vi "TIME_UPLOAD.vi"(8 "error in (no error)":errorcluster, 10 "Cluster":T2={"IP Address"=["", "", "", "", "", "", "", "", "", ""], "Machine name"=["", "", "", "", "", "", "", "", "", ""], "Station number"=["", "", "", "", "", "", "", "", "", ""], "Product List"=[], "Recipe_upload_history path"=path "", "reference"=refnum, "appended array"=[]}, 11 "CtlRef":refnum<vi>) -> (0 "error out":errorcluster, 3 "TIME DATA":i32[](array[numeric]), 5 "Time day":string[](array[string]))   [LabVIEW 2017]
uses:
  Controls/cluster.ctl
  <vilib>/addons/database/Connection.llb/Conn ObjectReference.ctl
  <vilib>/Utility/miscctls.llb/LVDateTimeRec.ctl
  <vilib>/addons/database/NI_Database_API.lvlib
panel:
  out "date time rec":T1
  in  "DAY 1":timestamp format="%<%X\n%x>T"
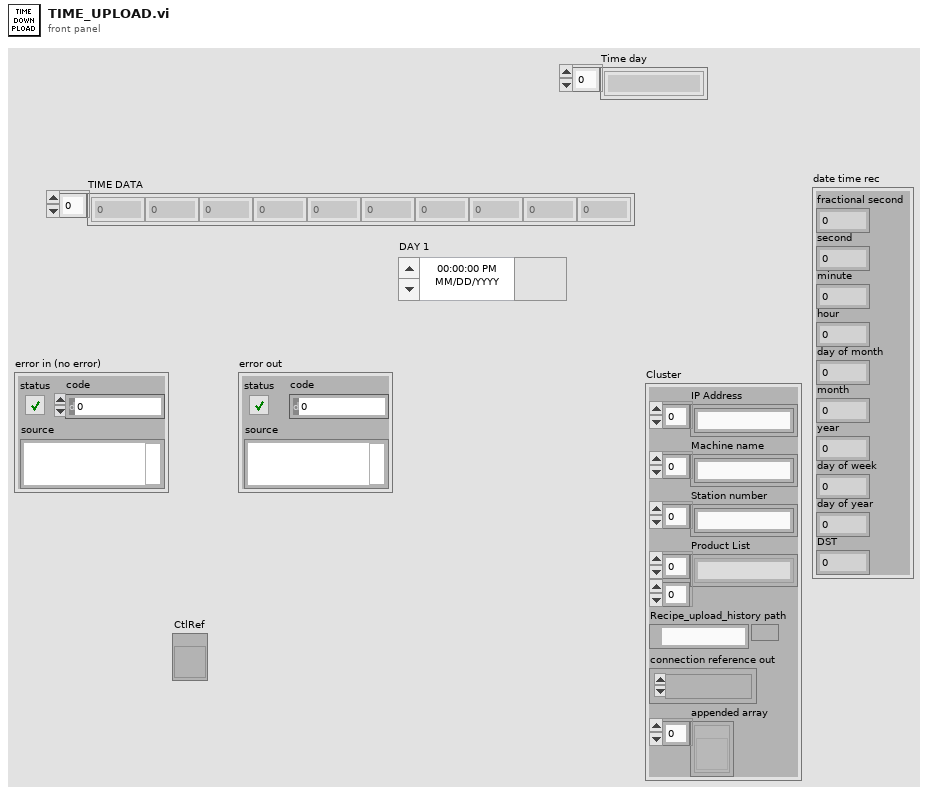
[diagram p1: front panel]
types:
  T1 = typedef "LVDateTimeRec.ctl" = cluster{"fractional second":dbl, "second":i32, "minute":i32, "hour":i32, "day of month":i32, "month":i32, "year":i32, "day of week":i32, "day of year":i32, "DST":i32}
  T2 = typedef "cluster.ctl" = cluster{"IP Address":string[], "Machine name":string[], "Station number":string[], "Product List":string[][], "Recipe_upload_history path":path, "reference":T3, "appended array":refnum<vi>[]}
  T3 = typedef "NI_Database_API.lvlib/Conn ObjectReference.ctl" = refnum<k1>
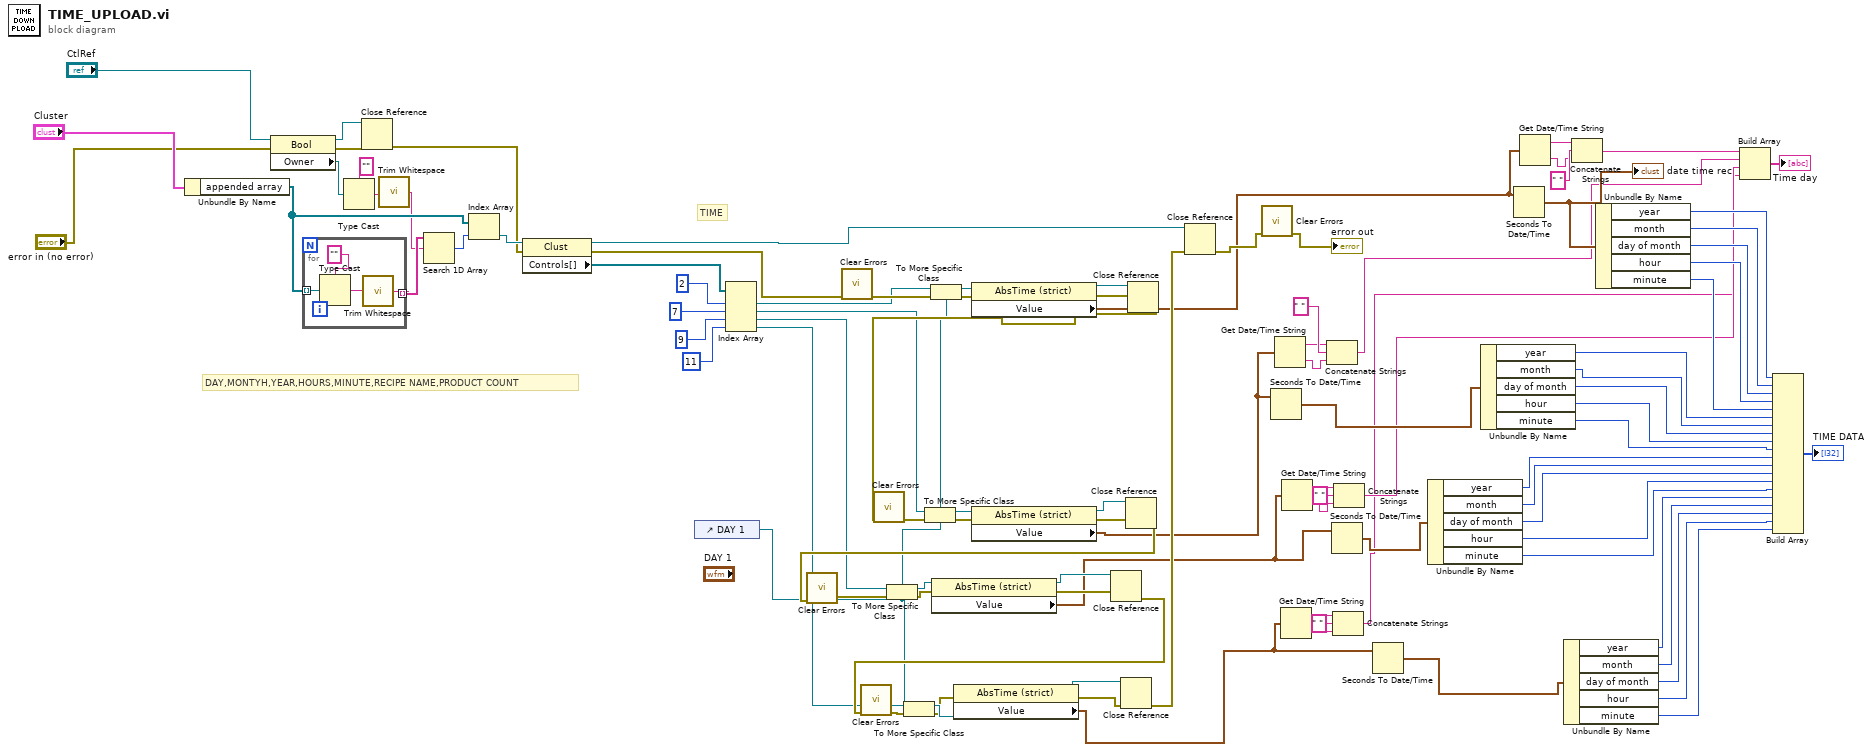
[diagram p0: block diagram]
diagram:
  # "DAY,MONTYH,YEAR,HOURS,MINUTE,RECIPE NAME,PRODUCT COUNT"
  # "TIME"
  n1 = Unbundle By Name("Cluster") -> ("appended array"=w61:refnum<vi>[])
  n2 = property class="Bool"(reference="CtlRef", error in="error in (no error)") -> (reference out=w53:refnum<vi>, error out=w54:errorcluster, "Owner"=w57:refnum<vi>)
  n3 = for {
    tunnel: w61 -> [w102] mode=indexing
    tunnel: [w99] -> w59 mode=indexing
    n4 = Type Cast(type="" ("String"), x=w102) -> (*(type *) &x=w100:string)
    n5 = call <vilib>:"Trim Whitespace.vi"("string"=w100) -> ("trimmed string"=w99:string)  [unwired: 1 in]
  }
  n6 = Type Cast(type="", x=w57) -> (*(type *) &x=w56:string)
  n7 = Close Reference(reference=w53, error in (no error)=w54) -> (error out=w49:errorcluster)
  n8 = call <vilib>:"Trim Whitespace.vi"("string"=w56) -> ("trimmed string"=w58:string)  [unwired: 1 in]
  n9 = Search 1D Array(1D array=w59, element=w58) -> (index of element=w60:i32)  [unwired: 1 in]
  n10 = Index Array(array=w61, index=w60) -> (element=w50:refnum<vi>)
  n11 = property class="Clust"(reference=w50, error in=w49) -> (reference out=w96:refnum<vi>, error out=w97:errorcluster, "Controls[]"=w94:refnum<vi>[])
  n12 = control-ref of="DAY 1"() -> (w63:refnum<vi>)
  n13 = Index Array(array=w94, index #1=2 ("index"), index #2=7 ("index"), index #3=9 ("index"), index #4=11 ("index")) -> (element #1=w67:refnum<vi>, element #2=w71:refnum<vi>, element #3=w76:refnum<vi>, element #4=w83:refnum<vi>)
  n14 = call <vilib>:"Clear Errors.vi"("error in (no error)"=w97) -> ("error out"=w70:errorcluster)  [unwired: 5 in, 1 out]
  n15 = To More Specific Class(target class=w63, reference=w67, error in=w70) -> (specific class reference=w68:refnum<vi>, error out=w69:errorcluster)
  n16 = property class="AbsTime (strict)"(reference=w68, error in=w69) -> (reference out=w86:refnum<vi>, error out=w95:errorcluster, "Value"=w21:timestamp)
  n17 = Close Reference(reference=w86, error in (no error)=w95) -> (error out=w89:errorcluster)
  n18 = call <vilib>:"Clear Errors.vi"("error in (no error)"=w89) -> ("error out"=w74:errorcluster)  [unwired: 5 in, 1 out]
  n19 = To More Specific Class(target class=w63, reference=w71, error in=w74) -> (specific class reference=w72:refnum<vi>, error out=w73:errorcluster)
  n20 = property class="AbsTime (strict)"(reference=w72, error in=w73) -> (reference out=w85:refnum<vi>, error out=w92:errorcluster, "Value"=w15:timestamp)
  n21 = Close Reference(reference=w85, error in (no error)=w92) -> (error out=w88:errorcluster)
  n22 = call <vilib>:"Clear Errors.vi"("error in (no error)"=w88) -> ("error out"=w77:errorcluster)  [unwired: 5 in, 1 out]
  n23 = To More Specific Class(target class=w63, reference=w76, error in=w77) -> (specific class reference=w75:refnum<vi>, error out=w78:errorcluster)
  n24 = property class="AbsTime (strict)"(reference=w75, error in=w78) -> (reference out=w84:refnum<vi>, error out=w91:errorcluster, "Value"=w12:timestamp)
  n25 = Close Reference(reference=w84, error in (no error)=w91) -> (error out=w87:errorcluster)
  n26 = call <vilib>:"Clear Errors.vi"("error in (no error)"=w87) -> ("error out"=w80:errorcluster)  [unwired: 5 in, 1 out]
  n27 = To More Specific Class(target class=w63, reference=w83, error in=w80) -> (specific class reference=w81:refnum<vi>, error out=w79:errorcluster)
  n28 = property on="Property Node" class="AbsTime (strict)"(reference=w81, error in=w79) -> (reference out=w82:refnum<vi>, error out=w62:errorcluster, "Value"=w10:timestamp)
  n29 = Close Reference(reference=w82, error in (no error)=w62) -> (error out=w90:errorcluster)
  n30 = Close Reference(reference=w96, error in (no error)=w90) -> (error out=w47:errorcluster)
  n31 = call <vilib>:"Clear Errors.vi"("error in (no error)"=w47) -> ("error out"=→"error out":errorcluster)  [unwired: 5 in, 1 out]
  n32 = Seconds To Date/Time(time stamp (now)=w15) -> (date time rec=w40:T1)  [unwired: 1 in]
  n33 = Get Date/Time String(seconds (now)=w15) -> (date string=w4:string, time string=w17:string)  [unwired: 2 in]
  n34 = Get Date/Time String(seconds (now)=w10) -> (date string=w2:string, time string=w1:string)  [unwired: 2 in]
  n35 = Get Date/Time String(seconds (now)=w12) -> (date string=w3:string, time string=w13:string)  [unwired: 2 in]
  n36 = Concatenate Strings(w4, " " ("string"), w17) -> (w8:string)
  n37 = Seconds To Date/Time(time stamp (now)=w12) -> (date time rec=w34:T1)  [unwired: 1 in]
  n38 = Concatenate Strings(w2, " " ("string"), w1) -> (w6:string)
  n39 = Concatenate Strings(w3, " " ("string"), w13) -> (w7:string)
  n40 = Seconds To Date/Time(time stamp (now)=w10) -> (date time rec=w28:T1)  [unwired: 1 in]
  n41 = Unbundle By Name(w34) -> ("year"=w33:i32, "month"=w32:i32, "day of month"=w31:i32, "hour"=w30:i32, "minute"=w29:i32)
  n42 = Unbundle By Name(w40) -> ("year"=w39:i32, "month"=w38:i32, "day of month"=w37:i32, "hour"=w36:i32, "minute"=w35:i32)
  n43 = Seconds To Date/Time(time stamp (now)=w21) -> (date time rec=w22:T1)  [unwired: 1 in]
  "date time rec" <- w22
  n44 = Get Date/Time String(seconds (now)=w21) -> (date string=w20:string, time string=w18:string)  [unwired: 2 in]
  n45 = Unbundle By Name(w28) -> ("year"=w27:i32, "month"=w26:i32, "day of month"=w25:i32, "hour"=w24:i32, "minute"=w23:i32)
  n46 = Concatenate Strings(w20, " " ("string"), w18) -> (w9:string)
  n47 = Unbundle By Name(w22) -> ("year"=w45:i32, "month"=w44:i32, "day of month"=w43:i32, "hour"=w42:i32, "minute"=w41:i32)
  n48 = Build Array(w9, w8, w7, w6) -> (→"Time day":string[])
  n49 = Build Array(w45, w44, w43, w42, w41, w39, w38, w37, w36, w35, w33, w32, w31, w30, w29, w27, w26, w25, w24, w23) -> (→"TIME DATA":i32[])
